vi "Send Alpha Task.vi"(7 "Message Priority (Normal)":T1=enum."Normal", 8 "error in (no error)":errorcluster, 10 "Data":i32, 11 "Message Enqueuer":refnum<class "Message Enqueuer.lvclass">) -> (0 "error out":errorcluster)   [LabVIEW 2026, in "Alpha Actor.lvlib" / "Alpha Task Msg.lvclass"]
uses:
  Alpha Task Msg.lvclass
  <vilib>/ActorFramework/Message Enqueuer/Message Enqueuer.lvclass
  <vilib>/ActorFramework/Message Enqueuer/Message Priority.ctl
  Alpha Task Msg.lvclass/Alpha Task Msg.ctl
  <vilib>/ActorFramework/Message Enqueuer/Message Enqueuer.lvclass/Message Enqueuer.ctl
  <vilib>/ActorFramework/Message Priority Queue/Priority Enqueue.vi
  C:/Program Files (x86)/National Instruments/LabVIEW 2026/vi.lib/ActorFramework/Message/Message.lvclass
  C:/git/CI-Automation/Source/Alpha Actor/Alpha Task Msg/Alpha Task Msg.lvclass
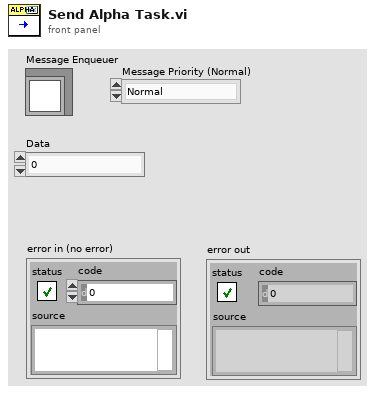
[diagram p1: front panel]
types:
  T1 = typedef "Actor Framework.lvlib/Message Enqueuer.lvclass/Message Priority.ctl" = enum16{"Low", "Normal", "High"}
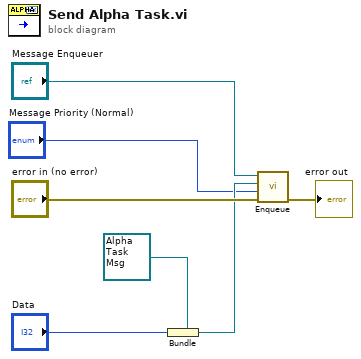
[diagram p0: block diagram]
diagram:
  n1 = Bundle(cluster=refnum<class "Alpha Task Msg.lvclass"> refnum ("Object"), "Data") -> (w3:refnum<class "Alpha Task Msg.lvclass">)
  n2 = call <vilib>:"Enqueue.vi"("error in (no error)"="error in (no error)", "Message Priority (Normal)"="Message Priority (Normal)", "Message"=w3, "Message Enqueuer in"="Message Enqueuer") -> ("error out"=→"error out":errorcluster)  [unwired: 6 in, 1 out]
